vi "MTCDT AP Slot Tests.vi"() -> ()   [LabVIEW 2024]
uses:
  AP slots to test.ctl
  Global 2.vi
panel:
  out "CMD line args":string[](array[string])
  in  "Save to log file (N)":bool
  in  "Loops":u32=1 min=1 step=1
  in  "Slot":T1=enum."AP1 and AP2"
  out "All Passed?":bool
  in  "VISA resource name":refnum<visa-resource-name>="COM5"
  out "error out":errorcluster
  in  "error in (no error)":errorcluster
  in  "Start":bool
  out "Test Log":string
  # "MTCDT AP Slot Tests"
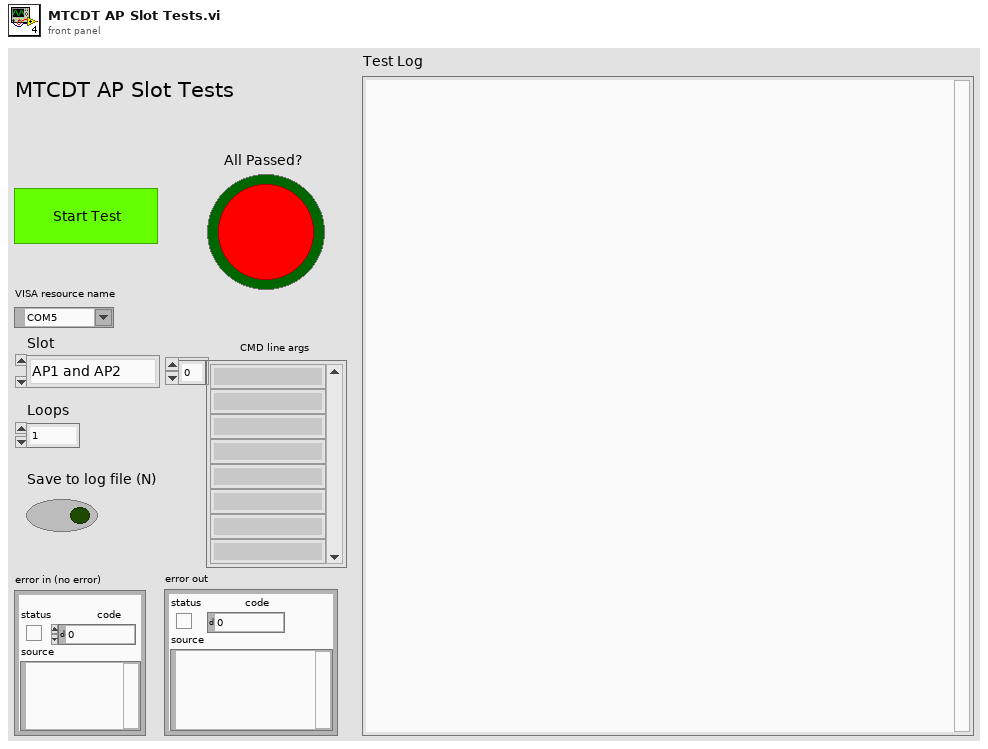
[diagram p1: front panel]
types:
  T1 = typedef "AP slots to test.ctl" = enum16{"Select Slot", "AP1", "AP2", "AP1 and AP2"}
  T2 = enum16{"open", "replace", "create", "open or create", "replace or create", "replace or create with confirmation"}
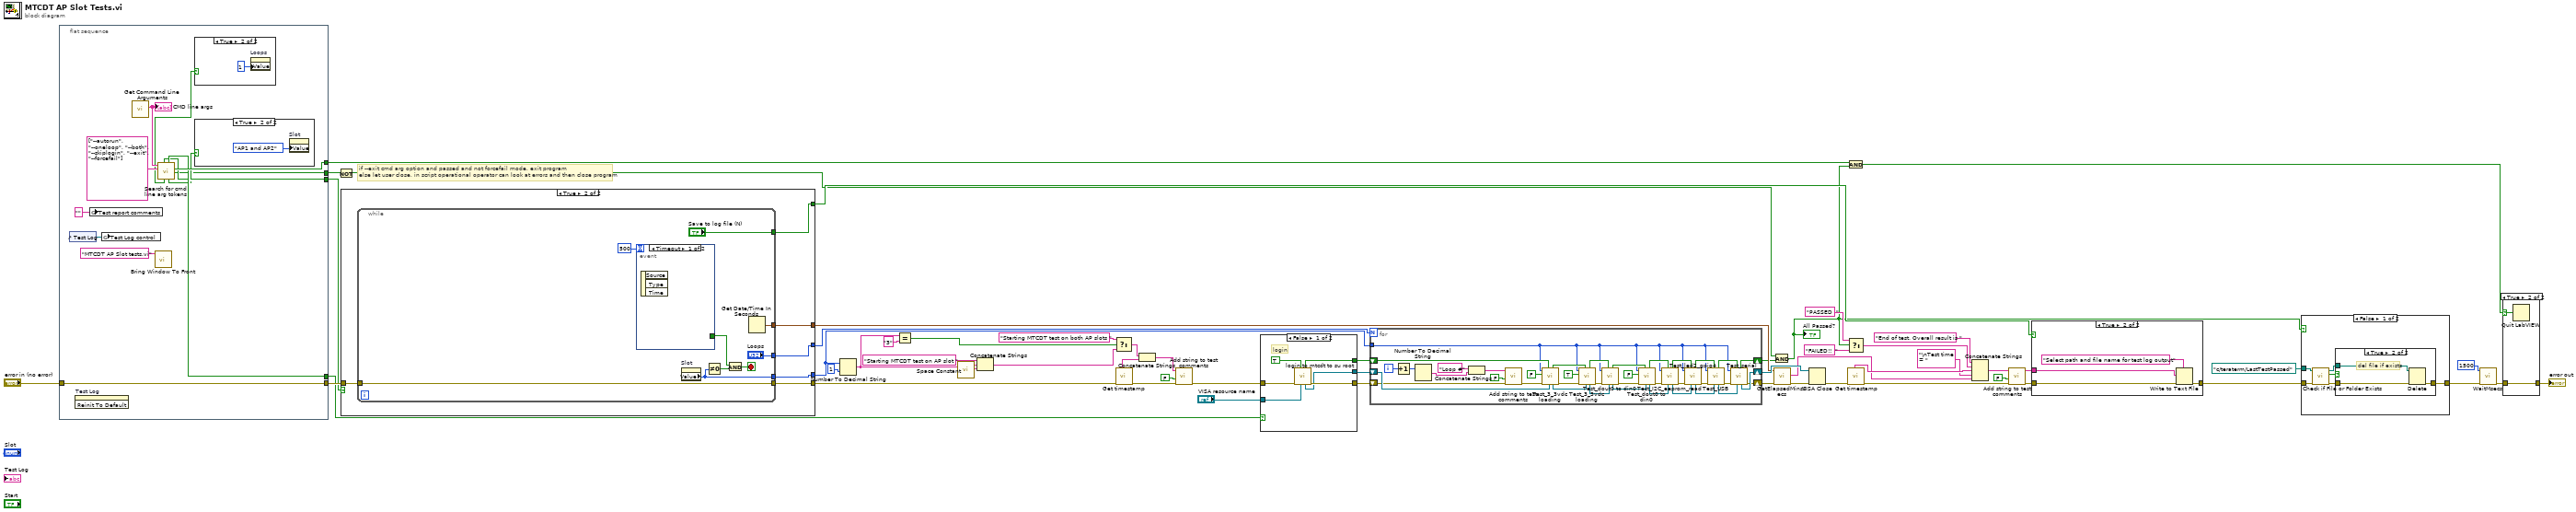
[diagram p0: block diagram]
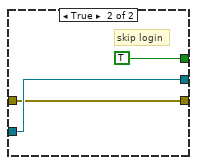
[diagram p3: hidden frame]
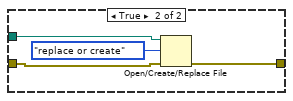
[diagram p5: hidden frame]
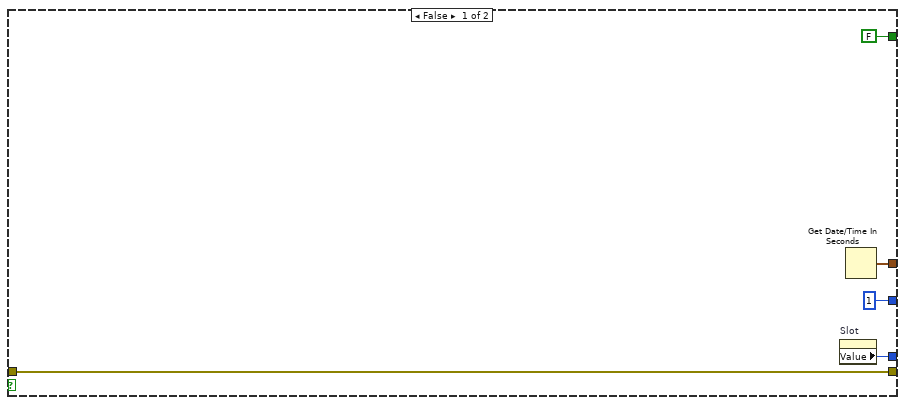
[diagram p6: hidden frame]
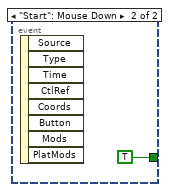
[diagram p7: hidden frame]
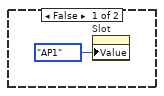
[diagram p9: hidden frame]
diagram:
  # "if --exit cmd arg option and passed and not forcefail mode, exit program\nelse let user close, in script operational operator can look at errors and then close program"
  n1 = flat-sequence {
    tunnel: [w67] -> w55
    tunnel: "error in (no error)" -> [w67]
    tunnel: [w58] -> w14
    tunnel: [w59] -> w11
    tunnel: [w60] -> w2
    tunnel: [w56] -> w6
    frame #0 {
      n2 = control-ref of="Test Log"() -> (w66:refnum<vi>)
      n3 = invoke on="Test Log" class="Str" method="Reinit To Default"() -> ()  [unwired: 3 in, 3 out]
      n4 = global write "Global 2.vi" "Test report comments"("" ("Test report comments")) -> ()
      n5 = global write "Global 2.vi" "Test Log control"(w66) -> ()
      n6 = call <vilib>:"Get Command Line Arguments.vi"() -> ("arguments"=w64:string[])  [unwired: 9 in, 2 out]
      "CMD line args" <- w64
      n7 = call "Bring Window To Front.vi"("Window Name"="MTCDT AP Slot tests.vi") -> ()  [unwired: 8 in, 3 out]
      n8 = call "Search for cmd line arg tokens.vi"("look for tokens"=string[] ["--autorun", "--oneloop", "--both", "--skiplogin", "--exit", "--forcefail"], "table"=w64) -> ("[5]"=w56:bool, "[4]"=w60:bool, "[2]"=w57:bool, "[3]"=w59:bool, "[1]"=w61:bool, "[0]"=w58:bool)  [unwired: 2 in, 2 out]
      n9 = case shown="True" w61 {
        frame False {
        }
        frame True {
          n10 = property on="Loops" class="DigNum (strict)"("Value"=u32 1 ("Loops")) -> ()  [unwired: 2 in, 2 out]
        }
      }
      n11 = case shown="True" w57 {
        frame False {
          n12 = property on="Slot" class="Enum (strict)"("Value"=AP_slots_to_test."AP1" ("Slot")) -> ()  [unwired: 2 in, 2 out]
        }
        frame True {
          n13 = property on="Slot" class="Enum (strict)"("Value"=AP_slots_to_test."AP1 and AP2" ("Slot")) -> ()  [unwired: 2 in, 2 out]
        }
      }
    }
  }
  n14 = Not(x=w6) -> (.not. x?=w4:bool)
  n15 = case shown="True" w14 {
    tunnel: w55 -> [w71 w81]
    tunnel: [w72 w80] -> w33
    tunnel: [u32 1 ("Loops") w79] -> w32
    tunnel: [FALSE ("Save to log file (N)") w78] -> w30
    tunnel: [w71 w77] -> w27
    tunnel: [w75 w76] -> w17
    frame False {
      n16 = property on="Slot" class="Enum (strict)"() -> ("Value"=w72:T1)  [unwired: 2 in, 2 out]
      n17 = Get Date/Time In Seconds() -> (seconds since 1Jan1904=w75:timestamp)
    }
    frame True {
      n18 = while {
        tunnel: [w89] -> w77
        tunnel: w81 -> [w89]
        tunnel: [w87] -> w80
        tunnel: ["Loops"] -> w79
        tunnel: ["Save to log file (N)"] -> w78
        tunnel: [w82] -> w76
        stop <- w85 stop-if-true
        n19 = event shown="[0] Timeout" {
          selector: _ -> [_ _]
          dyn-events: _ -> [_ _]
          timeout: 500 -> [_ _]
          tunnel: [_ TRUE] -> w88
          event Timeout {
            n20 = event-data() -> ()  [unwired: 1 in, 3 out]
          }
          event "Start": Mouse Down {
            n21 = event-data() -> ()  [unwired: 1 in, 8 out]
          }
        }
        n22 = property on="Slot" class="Enum (strict)"() -> ("Value"=w87:T1)  [unwired: 2 in, 2 out]
        n23 = Not Equal To 0?(x=w87) -> (x != 0?=w86:bool)
        n24 = And(x=w88, y=w86) -> (x .and. y?=w85:bool)
        n25 = Get Date/Time In Seconds() -> (seconds since 1Jan1904=w82:timestamp)
      }
    }
  }
  n26 = Number To Decimal String(number=w33, width (-)=i16 1) -> (decimal integer string=w35:string)
  n27 = Equal?(x=w35, y="3") -> (x = y?=w38:bool)
  n28 = call <vilib>:"Space Constant.vi"() -> ("String"=w20:string)
  n29 = Concatenate Strings("Starting MTCDT test on AP slot " ("Comments"), w35, w20) -> (w34:string)
  n30 = Select(t="Starting MTCDT test on both AP slots " ("Comments"), s=w38, f=w34) -> (s? t:f=w28:string)
  n31 = call "Get timestamp.vi"("error in (no error)"=w27) -> ("error out"=w26:errorcluster, "Date_time_for_filenames"=w25:string)  [unwired: 2 in, 7 out]
  n32 = Concatenate Strings(w28, w25) -> (w24:string)
  n33 = call "Add string to test comments.vi"("error in (no error)"=w26, "New Section (y)?"=FALSE, "Comments"=w24) -> ("error out"=w48:errorcluster)  [unwired: 7 in, 1 out]
  n34 = case shown="False" w11 {
    tunnel: [w97 w99] -> w53
    tunnel: "VISA resource name" -> [w96 w100]
    tunnel: [w95 TRUE ("Passed?")] -> w51
    tunnel: [w94 w100] -> w50
    tunnel: w48 -> [w92 w99]
    frame False {
      # "login"
      n35 = call "login to mtcdt to su root.vi"("VISA resource name"=w96, "Passed so far?"=TRUE, "error in (no error)"=w92) -> ("error out"=w97:errorcluster, "VISA resource name out"=w94:refnum<visa-resource-name>, "Passed?"=w95:bool)  [unwired: 4 in, 2 out]
    }
    frame True {
      # "skip login"
    }
  }
  n36 = for {
    N: w32 -> [_]
    tunnel: w33 -> [w101]
    shift-right: [w112] -> w19
    shift-left: w53 -> [w109]
    shift-right: [w113] -> w5
    shift-left: w51 -> [w136]
    shift-right: [w116] -> w41
    shift-left: w50 -> [w135]
    i -> [w108]
    n37 = Increment(x=w108) -> (x+1=w107:i32)
    n38 = Number To Decimal String(number=w107) -> (decimal integer string=w105:string)  [unwired: 1 in]
    n39 = Concatenate Strings("Loop #" ("string"), w105) -> (w104:string)
    n40 = call "Add string to test comments.vi"("error in (no error)"=w109, "New Section (y)?"=FALSE, "Comments"=w104) -> ("error out"=w102:errorcluster)  [unwired: 7 in, 1 out]
    n41 = call "Test_3_3vdc loading.vi"("VISA resource name"=w135, "Pass so far?"=w136, "error in (no error)"=w102, "3.3vdc Load ON (y)"=FALSE, "Slot"=w101) -> ("error out"=w126:errorcluster, "VISA resource name out"=w123:refnum<visa-resource-name>, "Passed?"=w125:bool)  [unwired: 2 in, 2 out]
    n42 = call "Test_3_3vdc loading.vi"("VISA resource name"=w123, "Pass so far?"=w125, "error in (no error)"=w126, "3.3vdc Load ON (y)"=TRUE, "Slot"=w101) -> ("error out"=w121:errorcluster, "VISA resource name out"=w122:refnum<visa-resource-name>, "Passed?"=w124:bool)  [unwired: 2 in, 2 out]
    n43 = call "Test_dout0 to din0.vi"("VISA resource name"=w122, "Passed so far?"=w124, "error in (no error)"=w121, "Slot"=w101) -> ("error out"=w138:errorcluster, "VISA resource name out"=w133:refnum<visa-resource-name>, "Passed?"=w134:bool)  [unwired: 4 in, 1 out]
    n44 = call "Test_dout0 to din0.vi"("VISA resource name"=w133, "Passed so far?"=w134, "error in (no error)"=w138, "Dout0 ON (y)"=FALSE, "Slot"=w101) -> ("error out"=w132:errorcluster, "VISA resource name out"=w130:refnum<visa-resource-name>, "Passed?"=w131:bool)  [unwired: 3 in, 1 out]
    n45 = call "Test_I2C_eeprom_read.vi"("VISA resource name"=w130, "Passed so far?"=w131, "error in (no error)"=w132, "Slot"=w101) -> ("error out"=w129:errorcluster, "VISA resource name out"=w128:refnum<visa-resource-name>, "Passed?"=w115:bool)  [unwired: 4 in, 1 out]
    n46 = call "Test_led2_gpio4.vi"("VISA resource name"=w128, "Passed so far?"=w115, "error in (no error)"=w129, "Slot"=w101) -> ("error out"=w120:errorcluster, "VISA resource name out"=w119:refnum<visa-resource-name>, "Passed?"=w111:bool)  [unwired: 4 in, 1 out]
    n47 = call "Test_USB.vi"("VISA resource name"=w119, "Passed so far?"=w111, "error in (no error)"=w120, "Slot"=w101) -> ("error out"=w118:errorcluster, "VISA resource name out"=w117:refnum<visa-resource-name>, "Passed?"=w114:bool)  [unwired: 4 in, 1 out]
    n48 = call "Test_serial.vi"("VISA resource name"=w117, "Passed so far?"=w114, "error in (no error)"=w118, "Slot"=w101) -> ("error out"=w112:errorcluster, "VISA resource name out"=w116:refnum<visa-resource-name>, "Passed?"=w113:bool)  [unwired: 4 in, 1 out]
  }
  n49 = And(x=w4, y=w5) -> (x .and. y?=w3:bool)
  "All Passed?" <- w3
  n50 = call "GetElapsedMinsSecs.vi"("error in (no error)"=w19, "Op Start Time"=w17) -> ("error out"=w18:errorcluster, "ElapsedTime"=w15:string)  [unwired: 6 in, 2 out]
  n51 = VISA Close(VISA resource name=w41, error in (no error)=w18) -> (error out=w23:errorcluster)
  n52 = And(x=w2, y=w3) -> (x .and. y?=w1:bool)
  n53 = Select(t="PASSED  ", s=w3, f="FAILED!!  ") -> (s? t:f=w44:string)
  n54 = call "Get timestamp.vi"("error in (no error)"=w23) -> ("error out"=w21:errorcluster, "Date_time_for_filenames"=w22:string)  [unwired: 2 in, 7 out]
  n55 = Concatenate Strings("End of test. Overall result is " ("string"), w44, w22, "\nTest time = " ("string"), w15) -> (w43:string)
  n56 = call "Add string to test comments.vi"("error in (no error)"=w21, "New Section (y)?"=FALSE, "Comments"=w43) -> ("error out"=w29:errorcluster, "concatenated string"=w31:string)  [unwired: 7 in]
  n57 = case shown="True" w30 {
    tunnel: w31 -> [_ w142]
    tunnel: w29 -> [w139 w143]
    tunnel: [w139 w140] -> w13
    frame False {
    }
    frame True {
      n58 = Write to Text File(prompt (Choose or enter file path)="Select path and file name for test log output", text=w142, error in=w143) -> (error out=w140:errorcluster)  [unwired: 1 in, 2 out]
    }
  }
  n59 = case shown="False" w3 {
    tunnel: w13 -> [w149 w156]
    tunnel: [w145 w155] -> w9
    tunnel: path "c:/teraterm/LastTestPassed" ("file path (use dialog)") -> [w144 w154]
    frame False {
      n60 = call <vilib>:"Check if File or Folder Exists.vi"("error in (no error)"=w149, "path"=w144) -> ("error out"=w146:errorcluster, "file or folder exists?"=w148:bool, "dup path"=w147:path)  [unwired: 7 in]
      n61 = case shown="True" w148 {
        tunnel: w147 -> [_ w153]
        tunnel: w146 -> [w150 w152]
        tunnel: [w150 w151] -> w145
        frame False {
        }
        frame True {
          # "del file if exists"
          n62 = Delete(path (use dialog)=w153, error in=w152) -> (error out=w151:errorcluster)  [unwired: 3 in, 2 out]
        }
      }
    }
    frame True {
      n63 = Open/Create/Replace File(file path (use dialog)=w154, error in=w156, operation (0:open)=T2."replace or create") -> (error out=w155:errorcluster)  [unwired: 3 in, 2 out]
    }
  }
  n64 = call "WaitMsecs.vi"("error in (no error)"=w9, "Wait Msecs"=u32 1500) -> ("error out"=w8:errorcluster)  [unwired: 9 in]
  n65 = case shown="True" w1 {
    selector: w1 -> [_ w159]
    tunnel: [w158 w160] -> w10
    tunnel: w8 -> [w158 w160]
    frame False {
    }
    frame True {
      n66 = Quit LabVIEW(quit? (T)=w159) -> ()
    }
  }
  "error out" <- w10
